vi "Write Auto Range.vi"(8 "error in (no error)":errorcluster, 10 "Auto Range":bool, 11 "3446X in":refnum<class "3446X.lvclass">) -> (0 "error out":errorcluster, 3 "3446X out":refnum<class "3446X.lvclass">)   [LabVIEW 2018, in "3446X.lvlib" / "3446X.lvclass"]
uses:
  3446X.lvclass
  3446X.lvclass/3446X.ctl
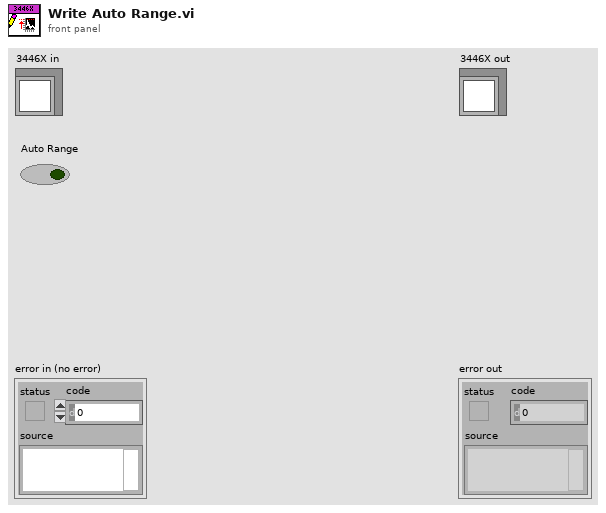
[diagram p1: front panel]
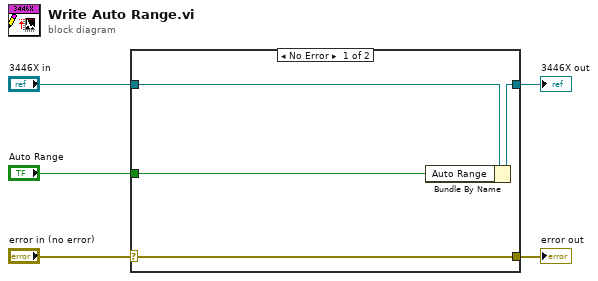
[diagram p0: block diagram]
diagram:
  n1 = case shown="No Error" "error in (no error)" {
    selector: "error in (no error)" -> [w9 w10]
    tunnel: [w9 w10] -> w4
    tunnel: [w7 w11] -> w2
    tunnel: "3446X in" -> [w8 w11]
    tunnel: "Auto Range" -> [w6 _]
    frame No Error {
      n2 = Bundle By Name(cluster=w8, "Auto Range"=w6) -> (w7:refnum<class "3446X.lvclass">)
    }
    frame Error {
    }
  }
  "error out" <- w4
  "3446X out" <- w2
